vi "Average.vi"(8 "Error In":errorcluster, 9 "Waveforms In":waveform(dbl)[](array[waveform]), 10 "Averaging":T1={"On"=FALSE, "Traces"=8, "Reset"=FALSE} {"Traces" min=1 max=200 step=1}) -> (0 "Error Out":errorcluster, 1 "Waveforms Out":waveform(dbl)[](array[waveform]), 2 "Traces":i32)   [LabVIEW 2016]
uses:
  Averaging.ctl
  Utilities/Circular Buffer Operations.ctl
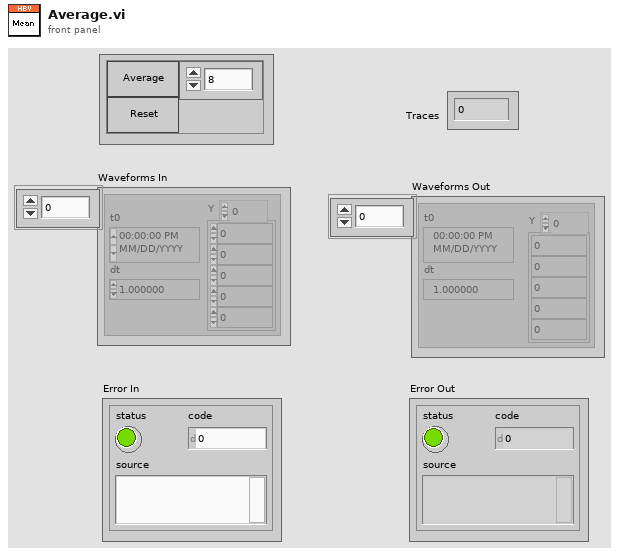
[diagram p1: front panel]
types:
  T1 = typedef "Averaging.ctl" = cluster{"On":bool, "Traces":i32, "Reset":bool}
  T2 = typedef "Circular Buffer Operations.ctl" = enum16{"Add data", "Reset"}
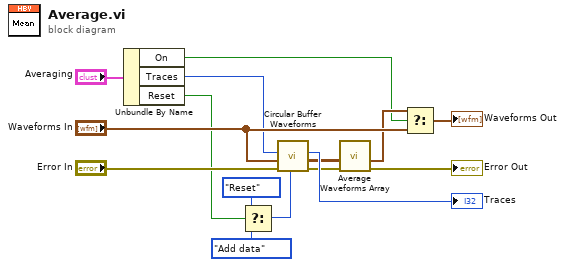
[diagram p0: block diagram]
diagram:
  n1 = Unbundle By Name("Averaging") -> ("On"=w6:bool, "Traces"=w5:i32, "Reset"=w4:bool)
  n2 = Select(t=Circular_Buffer_Operations."Reset" ("Action"), s=w4, f=Circular_Buffer_Operations."Add data" ("Action")) -> (s? t:f=w1:T2)
  n3 = call "Circular Buffer Waveforms.vi"("Action"=w1, "Error In"="Error In", "New Data"="Waveforms In", "Size"=w5) -> ("Error Out"=w8:errorcluster, "Buffer Out"=w9:waveform(dbl)[][], "Iterations"=→"Traces":i32)  [unwired: 4 in, 1 out]
  n4 = call "Average Waveforms Array.vi"("Error In"=w8, "Waveforms In"=w9) -> ("Error Out"=→"Error Out":errorcluster, "Averaged Waveforms"=w10:waveform(dbl)[])  [unwired: 8 in]
  n5 = Select(t=w10, s=w6, f="Waveforms In") -> (s? t:f=→"Waveforms Out":waveform(dbl)[])
